vi "Lab Panel V4.89.vi"() -> ()   [LabVIEW 2013] (continued)
                              tunnel: w5371 -> [_ w5375]
                              frame False {
                              }
                              frame True {
                                n2890 = Concatenate Strings("LA02-2 ", w5375) -> (w5378:string)
                                n2891 = One Button Dialog(message=w5378) -> ()  [unwired: 1 in, 1 out]
                              }
                            }
                          }
                          frame #4 {
                            n2892 = Greater?(x=w5380, y=w5383) -> (0:w5382:bool)
                            n2893 = case shown="True" w5382 {
                              tunnel: [w5384 0] -> w5379
                              tunnel: w5380 -> [w5384 _]
                              tunnel: w5381 -> [_ w5385]
                              frame False {
                              }
                              frame True {
                                n2894 = Concatenate Strings("LA03-1 ", w5385) -> (w5388:string)
                                n2895 = One Button Dialog(message=w5388) -> ()  [unwired: 1 in, 1 out]
                              }
                            }
                          }
                          frame #5 {
                            n2896 = Greater?(x=w5389, y=w5393) -> (0:w5392:bool)
                            n2897 = case shown="True" w5392 {
                              tunnel: [w5394 0] -> w5390
                              tunnel: w5389 -> [w5394 _]
                              tunnel: w5391 -> [_ w5395]
                              frame False {
                              }
                              frame True {
                                n2898 = Concatenate Strings("LA03-2 ", w5395) -> (w5398:string)
                                n2899 = One Button Dialog(message=w5398) -> ()  [unwired: 1 in, 1 out]
                              }
                            }
                          }
                          frame #6 {
                            n2900 = Greater?(x=w5400, y=w5403) -> (0:w5402:bool)
                            n2901 = case shown="True" w5402 {
                              tunnel: [w5404 0] -> w5399
                              tunnel: w5400 -> [w5404 _]
                              tunnel: w5401 -> [_ w5405]
                              frame False {
                              }
                              frame True {
                                n2902 = Concatenate Strings("LA04-1 ", w5405) -> (w5408:string)
                                n2903 = One Button Dialog(message=w5408) -> ()  [unwired: 1 in, 1 out]
                              }
                            }
                          }
                          frame #7 {
                            n2904 = Greater?(x=w5410, y=w5413) -> (0:w5412:bool)
                            n2905 = case shown="True" w5412 {
                              tunnel: [w5414 0] -> w5409
                              tunnel: w5410 -> [w5414 _]
                              tunnel: w5411 -> [_ w5415]
                              frame False {
                              }
                              frame True {
                                n2906 = Concatenate Strings("LA04-2 ", w5415) -> (w5418:string)
                                n2907 = One Button Dialog(message=w5418) -> ()  [unwired: 1 in, 1 out]
                              }
                            }
                          }
                          frame #8 {
                            n2908 = Greater?(x=w5420, y=w5423) -> (0:w5422:bool)
                            n2909 = case shown="True" w5422 {
                              tunnel: [w5424 0] -> w5419
                              tunnel: w5420 -> [w5424 _]
                              tunnel: w5421 -> [_ w5425]
                              frame False {
                              }
                              frame True {
                                n2910 = Concatenate Strings("LA05-1 ", w5425) -> (w5428:string)
                                n2911 = One Button Dialog(message=w5428) -> ()  [unwired: 1 in, 1 out]
                              }
                            }
                          }
                          frame #9 {
                            n2912 = Greater?(x=w5430, y=w5433) -> (0:w5432:bool)
                            n2913 = case shown="True" w5432 {
                              tunnel: [w5434 0] -> w5429
                              tunnel: w5430 -> [w5434 _]
                              tunnel: w5431 -> [_ w5435]
                              frame False {
                              }
                              frame True {
                                n2914 = Concatenate Strings("LA05-2 ", w5435) -> (w5438:string)
                                n2915 = One Button Dialog(message=w5438) -> ()  [unwired: 1 in, 1 out]
                              }
                            }
                          }
                        }
                        n2916 = Bundle By Name(cluster=w5337, "LAB01-1"=w5335, "LAB01-2"=w5333, "LAB02-1"=w5330, "LAB02-2"=w5327, "LAB03-1"=w5325, "LAB03-2"=w5324, "LAB04-1"=w5321, "LAB04-2"=w5319, "LAB05-1"=w5317, "LAB05-2"=w5315) -> (w5336:T8)
                        n2917 = local write "JIG RELAY CYCLES"(w5336) -> ()
                      }
                    }
                  }
                }
              }
            }
          }
          frame #19 {
            # "get temperature values"
            n2918 = local read "PANEL #"() -> (w5439:dbl)
            n2919 = local read "simulate"() -> (w5452:bool)
            n2920 = local read "Temp Test Cal"() -> (w5449:dbl)
            n2921 = stacked-sequence {
              seq-local: [w5453 _] -> [_ w5491]
              tunnel: w5452 -> [_ w5505]
              tunnel: T14 {"1  (A) cal"=1.0, "1 (V) cal"=1.0, "1 (PF) cal"=1.0, "1 (TL) cal"=1.0, "1 (TN) cal"=1.0, "2 (A) cal"=1.0, "2 (V) cal"=1.0, "2 (PF) cal"=1.0, "2 (TL) cal"=1.0, "2 (TN) cal"=1.0} ("CAL LAB01") -> [_ w5504]
              tunnel: w5450 -> [_ w5503]
              tunnel: w5449 -> [_ w5502]
              tunnel: w5448 -> [_ w5501]
              tunnel: w5447 -> [_ w5500]
              tunnel: w5446 -> [_ w5499]
              tunnel: w5445 -> [_ w5498]
              tunnel: w5444 -> [_ w5497]
              tunnel: w5443 -> [_ w5496]
              tunnel: w5442 -> [_ w5495]
              tunnel: w5441 -> [_ w5494]
              tunnel: w5440 -> [_ w5493]
              tunnel: w5439 -> [_ w5492]
              frame #0 {
                n2922 = local read "Select COM port"() -> (w5456:refnum<visa-resource-name>)
                "COM port" <- w5456
                n2923 = global write "Global 1.vi" "tmp dly lps"("Temp Delay Lps") -> ()
                n2924 = global write "Global 1.vi" "dly value"("Temp Value") -> ()
                n2925 = global write "Global 1.vi" "COM port"(w5456) -> ()
                n2926 = local read "jig cycle"() -> (w5458:dbl)
                n2927 = local read "on loops"() -> (w5460:dbl)
                n2928 = Add(x=w5460, y=3) -> (x+y=w5461:dbl)
                n2929 = local read "PANEL #"() -> (w5457:dbl)
                n2930 = Equal?(x=w5458, y=w5461) -> (x = y?=w5453:bool)
                n2931 = case shown="True" w5453 {
                  tunnel: w5457 -> [_ w5465]
                  frame False {
                  }
                  frame True {
                    n2932 = local read "simulate"() -> (w5462:bool)
                    n2933 = case shown="1" w5465 {
                      tunnel: 1.0 -> [_ w5470 w5472 w5478 w5482 w5487]
                      tunnel: w5462 -> [_ w5466 w5471 w5476 w5483 w5486]
                      frame 0, Default {
                      }
                      frame 1 {
                        w5468 = FALSE
                        n2934 = call "sub vi - GET ALL TEMP v6.vi"("LA01-EN"=TRUE, "simulate"=w5466, "LA02-EN"=w5468, "LA03-EN"=w5468, "LA04-EN"=w5468, "LA05-EN"=w5468, "Gen Cal Value"=w5470) -> ("LA01 TEMP"=w5467:T24)  [unwired: 3 in, 5 out]
                        n2935 = local write "LAB01 TEMP"(w5467) -> ()
                      }
                      frame 2 {
                        w5473 = FALSE
                        n2936 = call "sub vi - GET ALL TEMP v6.vi"("LA01-EN"=w5473, "simulate"=w5471, "LA02-EN"=TRUE, "LA03-EN"=w5473, "LA04-EN"=w5473, "LA05-EN"=w5473, "Gen Cal Value"=w5472) -> ("LA02 TEMP"=w5475:T24)  [unwired: 3 in, 5 out]
                        n2937 = local write "LAB02 TEMP"(w5475) -> ()
                      }
                      frame 3 {
                        w5479 = FALSE
                        n2938 = call "sub vi - GET ALL TEMP v6.vi"("LA01-EN"=w5479, "simulate"=w5476, "LA02-EN"=w5479, "LA03-EN"=TRUE, "LA04-EN"=w5479, "LA05-EN"=w5479, "Gen Cal Value"=w5478) -> ("LA03 TEMP"=w5477:T24)  [unwired: 3 in, 5 out]
                        n2939 = local write "LAB03 TEMP"(w5477) -> ()
                      }
                      frame 4 {
                        w5484 = FALSE
                        n2940 = call "sub vi - GET ALL TEMP v6.vi"("LA01-EN"=w5484, "simulate"=w5483, "LA02-EN"=w5484, "LA03-EN"=w5484, "LA04-EN"=TRUE, "LA05-EN"=w5484, "Gen Cal Value"=w5482) -> ("LA04 TEMP"=w5481:T24)  [unwired: 3 in, 5 out]
                        n2941 = local write "LAB04 TEMP"(w5481) -> ()
                      }
                      frame 5 {
                        w5489 = FALSE
                        n2942 = call "sub vi - GET ALL TEMP v6.vi"("LA01-EN"=w5489, "simulate"=w5486, "LA02-EN"=w5489, "LA03-EN"=w5489, "LA04-EN"=w5489, "LA05-EN"=TRUE, "Gen Cal Value"=w5487) -> ("LA05 TEMP"=w5488:T24)  [unwired: 3 in, 5 out]
                        n2943 = local write "LAB05 TEMP"(w5488) -> ()
                      }
                    }
                    n2944 = local write "TEMP"(TRUE) -> ()
                  }
                }
              }
              frame #1 {
                n2945 = case shown="True" w5491 {
                  tunnel: w5505 -> [_ w5519]
                  tunnel: w5504 -> [_ w5518]
                  tunnel: w5503 -> [_ w5517]
                  tunnel: w5502 -> [_ w5516]
                  tunnel: w5501 -> [_ w5515]
                  tunnel: w5500 -> [_ w5514]
                  tunnel: w5499 -> [_ w5513]
                  tunnel: w5498 -> [_ w5512]
                  tunnel: w5497 -> [_ w5511]
                  tunnel: w5496 -> [_ w5510]
                  tunnel: w5495 -> [_ w5509]
                  tunnel: w5494 -> [_ w5508]
                  tunnel: w5493 -> [_ w5507]
                  tunnel: w5492 -> [_ w5506]
                  frame False {
                  }
                  frame True {
                    n2946 = case shown="1" w5506 {
                      tunnel: w5519 -> [_ w5532 w5577 w5622 w5667 w5712]
                      tunnel: w5518 -> [_ w5531 w5576 w5621 w5666 w5711]
                      tunnel: w5517 -> [_ w5529 _ _ _ _]
                      tunnel: w5516 -> [_ w5525 w5575 w5620 w5665 w5710]
                      tunnel: w5515 -> [_ w5520 _ _ _ _]
                      tunnel: w5514 -> [_ _ w5566 _ _ _]
                      tunnel: w5513 -> [_ _ w5565 _ _ _]
                      tunnel: w5512 -> [_ _ _ w5611 _ _]
                      tunnel: w5511 -> [_ _ _ w5610 _ _]
                      tunnel: w5510 -> [_ _ _ _ w5656 _]
                      tunnel: w5509 -> [_ _ _ _ w5655 _]
                      tunnel: w5508 -> [_ _ _ _ _ w5701]
                      tunnel: w5507 -> [_ _ _ _ _ w5700]
                      frame ..0 {
                      }
                      frame 1 {
                        n2947 = case shown="False" w5532 {
                          tunnel: [w5563 w5564] -> w5548
                          tunnel: w5531 -> [_ w5564]
                          frame False {
                            n2948 = local read "CAL LAB01"() -> (w5563:T14)
                          }
                          frame True {
                          }
                        }
                        n2949 = local read "LAB01 TEMP"() -> (w5538:T12)
                        n2950 = local read "TEMP LA01"() -> (w5539:T9)
                        n2951 = call "sub vi - temperature delay v2.vi"("temp values IN"=w5539, "temp signals"=w5538) -> ("T2-N"=w5534:dbl, "T2-L"=w5535:dbl, "T1-N"=w5536:dbl, "T1-L"=w5537:dbl, "temp values OUT"=w5533:T43)  [unwired: 5 in]
                        n2952 = Unbundle By Name(w5548) -> ("1 (TL) cal"=w5543:dbl, "1 (TN) cal"=w5542:dbl, "2 (TL) cal"=w5541:dbl, "2 (TN) cal"=w5540:dbl)  [unwired: 6 out]
                        n2953 = local write "TEMP LA01"(w5533) -> ()
                        n2954 = Multiply(x=w5537, y=w5543) -> (x*y=w5530:dbl)
                        n2955 = Multiply(x=w5536, y=w5542) -> (x*y=w5527:dbl)
                        n2956 = Multiply(x=w5535, y=w5541) -> (x*y=w5524:dbl)
                        n2957 = Multiply(x=w5534, y=w5540) -> (x*y=w5523:dbl)
                        n2958 = case shown="True" w5529 {
                          tunnel: w5530 -> [w5557 w5562]
                          tunnel: w5525 -> [_ w5560]
                          tunnel: [w5557 w5561] -> w5528
                          tunnel: w5527 -> [w5556 w5559]
                          tunnel: [w5556 w5558] -> w5526
                          frame False {
                          }
                          frame True {
                            n2959 = Multiply(x=w5560, y=w5559) -> (x*y=w5558:dbl)
                            n2960 = Multiply(x=w5560, y=w5562) -> (x*y=w5561:dbl)
                          }
                        }
                        n2961 = case shown="True" w5520 {
                          tunnel: w5524 -> [w5550 w5555]
                          tunnel: w5525 -> [_ w5553]
                          tunnel: [w5550 w5554] -> w5522
                          tunnel: w5523 -> [w5549 w5552]
                          tunnel: [w5549 w5551] -> w5521
                          frame False {
                          }
                          frame True {
                            n2962 = Multiply(x=w5553, y=w5552) -> (x*y=w5551:dbl)
                            n2963 = Multiply(x=w5553, y=w5555) -> (x*y=w5554:dbl)
                          }
                        }
                        n2964 = local read "SIG LAB01-2"() -> (w5545:T2)
                        n2965 = local read "SIG LAB01-1"() -> (w5547:T2)
                        n2966 = Bundle By Name(cluster=w5547, "Tmp Live"=w5528, "Tmp Neut"=w5526) -> (w5546:T2)
                        n2967 = Bundle By Name(cluster=w5545, "Tmp Live"=w5522, "Tmp Neut"=w5521) -> (w5544:T2)
                        n2968 = local write "SIG LAB01-1"(w5546) -> ()
                        n2969 = local write "SIG LAB01-2"(w5544) -> ()
                      }
                      frame 2 {
                        n2970 = case shown="True" w5577 {
                          tunnel: [w5608 w5609] -> w5593
                          tunnel: w5576 -> [_ w5609]
                          frame False {
                            n2971 = local read "CAL LAB02"() -> (w5608:T15)
                          }
                          frame True {
                          }
                        }
                        n2972 = local read "LAB02 TEMP"() -> (w5584:T12)
                        n2973 = local read "TEMP LA02"() -> (w5583:T9)
                        n2974 = call "sub vi - temperature delay v2.vi"("temp values IN"=w5583, "temp signals"=w5584) -> ("T2-N"=w5578:dbl, "T2-L"=w5579:dbl, "T1-N"=w5580:dbl, "T1-L"=w5581:dbl, "temp values OUT"=w5582:T43)  [unwired: 5 in]
                        n2975 = Unbundle By Name(w5593) -> ("1 (TL) cal"=w5588:dbl, "1 (TN) cal"=w5587:dbl, "2 (TL) cal"=w5586:dbl, "2 (TN) cal"=w5585:dbl)  [unwired: 6 out]
                        n2976 = local write "TEMP LA02"(w5582) -> ()
                        n2977 = Multiply(x=w5581, y=w5588) -> (x*y=w5574:dbl)
                        n2978 = Multiply(x=w5580, y=w5587) -> (x*y=w5573:dbl)
                        n2979 = Multiply(x=w5579, y=w5586) -> (x*y=w5570:dbl)
                        n2980 = Multiply(x=w5578, y=w5585) -> (x*y=w5569:dbl)
                        n2981 = case shown="True" w5566 {
                          tunnel: w5574 -> [w5602 w5607]
                          tunnel: w5575 -> [_ w5605]
                          tunnel: [w5602 w5606] -> w5572
                          tunnel: w5573 -> [w5601 w5604]
                          tunnel: [w5601 w5603] -> w5571
                          frame False {
                          }
                          frame True {
                            n2982 = Multiply(x=w5605, y=w5604) -> (x*y=w5603:dbl)
                            n2983 = Multiply(x=w5605, y=w5607) -> (x*y=w5606:dbl)
                          }
                        }
                        n2984 = case shown="True" w5565 {
                          tunnel: w5570 -> [w5595 w5600]
                          tunnel: w5575 -> [_ w5598]
                          tunnel: [w5595 w5599] -> w5568
                          tunnel: w5569 -> [w5594 w5597]
                          tunnel: [w5594 w5596] -> w5567
                          frame False {
                          }
                          frame True {
                            n2985 = Multiply(x=w5598, y=w5597) -> (x*y=w5596:dbl)
                            n2986 = Multiply(x=w5598, y=w5600) -> (x*y=w5599:dbl)
                          }
                        }
                        n2987 = local read "SIG LAB02-2"() -> (w5590:T2)
                        n2988 = local read "SIG LAB02-1"() -> (w5592:T2)
                        n2989 = Bundle By Name(cluster=w5592, "Tmp Live"=w5572, "Tmp Neut"=w5571) -> (w5591:T2)
                        n2990 = Bundle By Name(cluster=w5590, "Tmp Live"=w5568, "Tmp Neut"=w5567) -> (w5589:T2)
                        n2991 = local write "SIG LAB02-1"(w5591) -> ()
                        n2992 = local write "SIG LAB02-2"(w5589) -> ()
                      }
                      frame 3 {
                        n2993 = case shown="False" w5622 {
                          tunnel: [w5653 w5654] -> w5638
                          tunnel: w5621 -> [_ w5654]
                          frame False {
                            n2994 = local read "CAL LAB03"() -> (w5653:T14)
                          }
                          frame True {
                          }
                        }
                        n2995 = local read "TEMP LA03"() -> (w5628:T9)
                        n2996 = local read "LAB03 TEMP"() -> (w5629:T12)
                        n2997 = call "sub vi - temperature delay v2.vi"("temp values IN"=w5628, "temp signals"=w5629) -> ("T2-N"=w5623:dbl, "T2-L"=w5624:dbl, "T1-N"=w5625:dbl, "T1-L"=w5626:dbl, "temp values OUT"=w5627:T43)  [unwired: 5 in]
                        n2998 = Unbundle By Name(w5638) -> ("1 (TL) cal"=w5633:dbl, "1 (TN) cal"=w5632:dbl, "2 (TL) cal"=w5631:dbl, "2 (TN) cal"=w5630:dbl)  [unwired: 6 out]
                        n2999 = local write "TEMP LA03"(w5627) -> ()
                        n3000 = Multiply(x=w5626, y=w5633) -> (x*y=w5619:dbl)
                        n3001 = Multiply(x=w5625, y=w5632) -> (x*y=w5618:dbl)
                        n3002 = Multiply(x=w5624, y=w5631) -> (x*y=w5615:dbl)
                        n3003 = Multiply(x=w5623, y=w5630) -> (x*y=w5614:dbl)
                        n3004 = case shown="True" w5610 {
                          tunnel: w5615 -> [w5640 w5645]
                          tunnel: w5620 -> [_ w5643]
                          tunnel: [w5640 w5644] -> w5613
                          tunnel: w5614 -> [w5639 w5642]
                          tunnel: [w5639 w5641] -> w5612
                          frame False {
                          }
                          frame True {
                            n3005 = Multiply(x=w5643, y=w5642) -> (x*y=w5641:dbl)
                            n3006 = Multiply(x=w5643, y=w5645) -> (x*y=w5644:dbl)
                          }
                        }
                        n3007 = case shown="True" w5611 {
                          tunnel: w5619 -> [w5647 w5652]
                          tunnel: w5620 -> [_ w5650]
                          tunnel: [w5647 w5651] -> w5617
                          tunnel: w5618 -> [w5646 w5649]
                          tunnel: [w5646 w5648] -> w5616
                          frame False {
                          }
                          frame True {
                            n3008 = Multiply(x=w5650, y=w5649) -> (x*y=w5648:dbl)
                            n3009 = Multiply(x=w5650, y=w5652) -> (x*y=w5651:dbl)
                          }
                        }
                        n3010 = local read "SIG LAB03-2"() -> (w5635:T2)
                        n3011 = local read "SIG LAB03-1"() -> (w5637:T2)
                        n3012 = Bundle By Name(cluster=w5637, "Tmp Live"=w5617, "Tmp Neut"=w5616) -> (w5636:T2)
                        n3013 = Bundle By Name(cluster=w5635, "Tmp Live"=w5613, "Tmp Neut"=w5612) -> (w5634:T2)
                        n3014 = local write "SIG LAB03-1"(w5636) -> ()
                        n3015 = local write "SIG LAB03-2"(w5634) -> ()
                      }
                      frame 4 {
                        n3016 = case shown="False" w5667 {
                          tunnel: [w5698 w5699] -> w5683
                          tunnel: w5666 -> [_ w5699]
                          frame False {
                            n3017 = local read "CAL LAB04"() -> (w5698:T14)
                          }
                          frame True {
                          }
                        }
                        n3018 = local read "LAB04 TEMP"() -> (w5673:T12)
                        n3019 = local read "TEMP LA04"() -> (w5674:T9)
                        n3020 = call "sub vi - temperature delay v2.vi"("temp values IN"=w5674, "temp signals"=w5673) -> ("T2-N"=w5668:dbl, "T2-L"=w5669:dbl, "T1-N"=w5670:dbl, "T1-L"=w5671:dbl, "temp values OUT"=w5672:T43)  [unwired: 5 in]
                        n3021 = Unbundle By Name(w5683) -> ("1 (TL) cal"=w5678:dbl, "1 (TN) cal"=w5677:dbl, "2 (TL) cal"=w5676:dbl, "2 (TN) cal"=w5675:dbl)  [unwired: 6 out]
                        n3022 = local write "TEMP LA04"(w5672) -> ()
                        n3023 = Multiply(x=w5671, y=w5678) -> (x*y=w5664:dbl)
                        n3024 = Multiply(x=w5670, y=w5677) -> (x*y=w5663:dbl)
                        n3025 = Multiply(x=w5669, y=w5676) -> (x*y=w5660:dbl)
                        n3026 = Multiply(x=w5668, y=w5675) -> (x*y=w5659:dbl)
                        n3027 = case shown="True" w5655 {
                          tunnel: w5660 -> [w5685 w5690]
                          tunnel: w5665 -> [_ w5688]
                          tunnel: [w5685 w5689] -> w5658
                          tunnel: w5659 -> [w5684 w5687]
                          tunnel: [w5684 w5686] -> w5657
                          frame False {
                          }
                          frame True {
                            n3028 = Multiply(x=w5688, y=w5687) -> (x*y=w5686:dbl)
                            n3029 = Multiply(x=w5688, y=w5690) -> (x*y=w5689:dbl)
                          }
                        }
                        n3030 = case shown="True" w5656 {
                          tunnel: w5664 -> [w5692 w5697]
                          tunnel: w5665 -> [_ w5695]
                          tunnel: [w5692 w5696] -> w5662
                          tunnel: w5663 -> [w5691 w5694]
                          tunnel: [w5691 w5693] -> w5661
                          frame False {
                          }
                          frame True {
                            n3031 = Multiply(x=w5695, y=w5694) -> (x*y=w5693:dbl)
                            n3032 = Multiply(x=w5695, y=w5697) -> (x*y=w5696:dbl)
                          }
                        }
                        n3033 = local read "SIG LAB04-2"() -> (w5680:T2)
                        n3034 = local read "SIG LAB04-1"() -> (w5682:T2)
                        n3035 = Bundle By Name(cluster=w5682, "Tmp Live"=w5662, "Tmp Neut"=w5661) -> (w5681:T2)
                        n3036 = Bundle By Name(cluster=w5680, "Tmp Live"=w5658, "Tmp Neut"=w5657) -> (w5679:T2)
                        n3037 = local write "SIG LAB04-1"(w5681) -> ()
                        n3038 = local write "SIG LAB04-2"(w5679) -> ()
                      }
                      frame 5.. {
                        n3039 = case shown="False" w5712 {
                          tunnel: [w5743 w5744] -> w5728
                          tunnel: w5711 -> [_ w5744]
                          frame False {
                            n3040 = local read "CAL LAB05"() -> (w5743:T14)
                          }
                          frame True {
                          }
                        }
                        n3041 = local read "LAB05 TEMP"() -> (w5718:T12)
                        n3042 = local read "TEMP LA05"() -> (w5719:T9)
                        n3043 = call "sub vi - temperature delay v2.vi"("temp values IN"=w5719, "temp signals"=w5718) -> ("T2-N"=w5714:dbl, "T2-L"=w5715:dbl, "T1-N"=w5716:dbl, "T1-L"=w5717:dbl, "temp values OUT"=w5713:T43)  [unwired: 5 in]
                        n3044 = local write "TEMP LA05"(w5713) -> ()
                        n3045 = Unbundle By Name(w5728) -> ("1 (TL) cal"=w5720:dbl, "1 (TN) cal"=w5723:dbl, "2 (TL) cal"=w5722:dbl, "2 (TN) cal"=w5721:dbl)  [unwired: 6 out]
                        n3046 = Multiply(x=w5717, y=w5720) -> (x*y=w5709:dbl)
                        n3047 = Multiply(x=w5716, y=w5723) -> (x*y=w5708:dbl)
                        n3048 = Multiply(x=w5715, y=w5722) -> (x*y=w5705:dbl)
                        n3049 = Multiply(x=w5714, y=w5721) -> (x*y=w5704:dbl)
                        n3050 = case shown="True" w5700 {
                          tunnel: w5705 -> [w5730 w5735]
                          tunnel: w5710 -> [_ w5733]
                          tunnel: [w5730 w5734] -> w5703
                          tunnel: w5704 -> [w5729 w5732]
                          tunnel: [w5729 w5731] -> w5702
                          frame False {
                          }
                          frame True {
                            n3051 = Multiply(x=w5733, y=w5732) -> (x*y=w5731:dbl)
                            n3052 = Multiply(x=w5733, y=w5735) -> (x*y=w5734:dbl)
                          }
                        }
                        n3053 = case shown="True" w5701 {
                          tunnel: w5709 -> [w5737 w5742]
                          tunnel: w5710 -> [_ w5740]
                          tunnel: [w5737 w5741] -> w5707
                          tunnel: w5708 -> [w5736 w5739]
                          tunnel: [w5736 w5738] -> w5706
                          frame False {
                          }
                          frame True {
                            n3054 = Multiply(x=w5740, y=w5739) -> (x*y=w5738:dbl)
                            n3055 = Multiply(x=w5740, y=w5742) -> (x*y=w5741:dbl)
                          }
                        }
                        n3056 = local read "SIG LAB05-1"() -> (w5727:T2)
                        n3057 = Bundle By Name(cluster=w5727, "Tmp Live"=w5707, "Tmp Neut"=w5706) -> (w5726:T2)
                        n3058 = local read "SIG LAB05-2"() -> (w5725:T2)
                        n3059 = Bundle By Name(cluster=w5725, "Tmp Live"=w5703, "Tmp Neut"=w5702) -> (w5724:T2)
                        n3060 = local write "SIG LAB05-1"(w5726) -> ()
                        n3061 = local write "SIG LAB05-2"(w5724) -> ()
                      }
                    }
                  }
                }
              }
            }
          }
          frame #20 {
            # "write data to display panel"
            n3062 = global write "Global display 1.vi" "TEST 5-2"(w5779) -> ()
            n3063 = global write "Global display 1.vi" "TEST 4-2"(w5781) -> ()
            n3064 = global write "Global display 1.vi" "TEST 1-2"(w5787) -> ()
            n3065 = global write "Global display 1.vi" "TEST 3-1"(w5784) -> ()
            n3066 = global write "Global display 1.vi" "TEST 5-1"(w5780) -> ()
            n3067 = global write "Global display 1.vi" "TEST 1-1"(w5788) -> ()
            n3068 = global write "Global display 1.vi" "TEST 3-2"(w5783) -> ()
            n3069 = global write "Global display 1.vi" "TEST 4-1"(w5782) -> ()
            n3070 = global write "Global display 1.vi" "TEST 2-2"(w5785) -> ()
            n3071 = global write "Global display 1.vi" "TEST 2-1"(w5786) -> ()
            n3072 = global read "Global display 3.vi" "log 1-1"() -> (→"LOG LAB01-1":string)
            n3073 = global read "Global display 3.vi" "log 3-1"() -> (→"LOG LAB03-1":string)
            n3074 = global read "Global display 3.vi" "log 1-2"() -> (→"LOG LAB01-2":string)
            n3075 = property on="Tab Control 2" class="TabCtl (strict)"() -> ("Pages"=w5778:refnum<vi>[])  [unwired: 2 in, 2 out]
            n3076 = global read "Global display 3.vi" "log 2-1"() -> (→"LOG LAB02-1":string)
            n3077 = global read "Global display 3.vi" "log 2-2"() -> (→"LOG LAB02-2":string)
            n3078 = global read "Global display 3.vi" "log 4-2"() -> (→"LOG LAB04-2":string)
            n3079 = global read "Global display 3.vi" "log 5-2"() -> (→"LOG LAB05-2":string)
            n3080 = global read "Global display 3.vi" "log 5-1"() -> (→"LOG LAB05-1":string)
            n3081 = global read "Global display 3.vi" "log 4-1"() -> (→"LOG LAB04-1":string)
            n3082 = global read "Global display 3.vi" "log 3-2"() -> (→"LOG LAB03-2":string)
            n3083 = Index Array(array=w5778, index=8) -> (element=w5776:refnum<vi>)
            n3084 = property class="Page"(reference=w5776) -> ("PageVis"=w5775:bool)  [unwired: 1 in, 2 out]
            n3085 = global write "Global display 3.vi" "admin"(w5775) -> ()
            n3086 = local read "O/I  LAB05-2"() -> (w5829:bool)
            n3087 = local read "O/I  LAB05-1"() -> (w5830:bool)
            n3088 = local read "O/I  LAB03-2"() -> (w5833:bool)
            n3089 = local read "O/I  LAB04-2"() -> (w5831:bool)
            n3090 = local read "O/I  LAB04-1"() -> (w5832:bool)
            n3091 = local read "O/I  LAB03-1"() -> (w5834:bool)
            n3092 = local read "O/I  LAB01-2"() -> (w5837:bool)
            n3093 = local read "O/I  LAB01-1"() -> (w5838:bool)
            n3094 = local read "O/I  LAB02-1"() -> (w5836:bool)
            n3095 = local read "O/I  LAB02-2"() -> (w5835:bool)
            n3096 = global write "Global display 1.vi" "5-2 O/F"(w5829) -> ()
            n3097 = global write "Global display 1.vi" "5-1 O/F"(w5830) -> ()
            n3098 = global write "Global display 1.vi" "4-1 O/F"(w5832) -> ()
            n3099 = global write "Global display 1.vi" "4-2 O/F"(w5831) -> ()
            n3100 = global write "Global display 1.vi" "3-2 O/F"(w5833) -> ()
            n3101 = global write "Global display 1.vi" "3-1 O/F"(w5834) -> ()
            n3102 = global write "Global display 1.vi" "2-2 O/F"(w5835) -> ()
            n3103 = global write "Global display 1.vi" "2-1 O/F"(w5836) -> ()
            n3104 = global write "Global display 1.vi" "1-2 O/F"(w5837) -> ()
            n3105 = global write "Global display 1.vi" "1-1 O/F"(w5838) -> ()
            n3106 = local read "TEMP START LAB02-2"() -> (w5761:cluster{"TL":dbl, "TN":dbl})
            n3107 = local read "run lab05-2"() -> (w5819:bool)
            n3108 = local read "TEMP START LAB01-2"() -> (w5763:cluster{"TL":dbl, "TN":dbl})
            n3109 = local read "TEMP START LAB02-1"() -> (w5762:cluster{"TL":dbl, "TN":dbl})
            n3110 = local read "TEMP START LAB04-1"() -> (w5758:cluster{"TL":dbl, "TN":dbl})
            n3111 = local read "TEMP START LAB04-2"() -> (w5757:cluster{"TL":dbl, "TN":dbl})
            n3112 = local read "run lab04-1"() -> (w5822:bool)
            n3113 = local read "run lab04-2"() -> (w5821:bool)
            n3114 = local read "run lab05-1"() -> (w5820:bool)
            n3115 = local read "TEMP START LAB01-1"() -> (w5764:cluster{"TL":dbl, "TN":dbl})
            n3116 = local read "TEMP START LAB05-2"() -> (w5755:cluster{"TL":dbl, "TN":dbl})
            n3117 = local read "TEMP START LAB05-1"() -> (w5756:cluster{"TL":dbl, "TN":dbl})
            n3118 = local read "run lab03-2"() -> (w5823:bool)
            n3119 = local read "TEMP START LAB03-2"() -> (w5759:cluster{"TL":dbl, "TN":dbl})
            n3120 = local read "TEMP START LAB03-1"() -> (w5760:cluster{"TL":dbl, "TN":dbl})
            n3121 = local read "run lab02-1"() -> (w5826:bool)
            n3122 = local read "run lab03-1"() -> (w5824:bool)
            n3123 = local read "run lab01-2"() -> (w5827:bool)
            n3124 = local read "run lab02-2"() -> (w5825:bool)
            n3125 = local read "run lab01-1"() -> (w5828:bool)
            n3126 = global write "Global display 1.vi" "5-2 R/S"(w5819) -> ()
            n3127 = global write "Global display 1.vi" "5-1 R/S"(w5820) -> ()
            n3128 = global write "Global display 1.vi" "4-2 R/S"(w5821) -> ()
            n3129 = global write "Global display 1.vi" "4-1 R/S"(w5822) -> ()
            n3130 = global write "Global display 1.vi" "3-2 R/S"(w5823) -> ()
            n3131 = global write "Global display 1.vi" "1-2 R/S"(w5827) -> ()
            n3132 = global write "Global display 1.vi" "2-1 R/S"(w5826) -> ()
            n3133 = global write "Global display 1.vi" "3-1 R/S"(w5824) -> ()
            n3134 = global write "Global display 1.vi" "2-2 R/S"(w5825) -> ()
            n3135 = global write "Global display 1.vi" "1-1 R/S"(w5828) -> ()
            n3136 = global write "Global display 3.vi" "TEMP ST 05-2"(w5755) -> ()
            n3137 = global write "Global display 3.vi" "TEMP ST 05-1"(w5756) -> ()
            n3138 = global write "Global display 3.vi" "TEMP ST 03-2"(w5759) -> ()
            n3139 = global write "Global display 3.vi" "TEMP ST 04-2"(w5757) -> ()
            n3140 = global write "Global display 3.vi" "TEMP ST 01-1"(w5764) -> ()
            n3141 = global write "Global display 3.vi" "TEMP ST 01-2"(w5763) -> ()
            n3142 = global write "Global display 3.vi" "TEMP ST 04-1"(w5758) -> ()
            n3143 = global write "Global display 3.vi" "TEMP ST 02-1"(w5762) -> ()
            n3144 = global write "Global display 3.vi" "TEMP ST 02-2"(w5761) -> ()
            n3145 = global write "Global display 3.vi" "TEMP ST 03-1"(w5760) -> ()
            n3146 = local read "DISP LAB04-2"() -> (w5811:T4)
            n3147 = local read "DISP LAB05-1"() -> (w5810:T4)
            n3148 = local read "DISP LAB04-1"() -> (w5812:T4)
            n3149 = local read "DISP LAB05-2"() -> (w5809:T4)
            n3150 = local read "DISP LAB03-1"() -> (w5814:T4)
            n3151 = local read "DISP LAB03-2"() -> (w5813:T4)
            n3152 = local read "DISP LAB01-2"() -> (w5817:T4)
            n3153 = local read "DISP LAB02-1"() -> (w5816:T4)
            n3154 = local read "DISP LAB02-2"() -> (w5815:T4)
            n3155 = local read "DISP LAB01-1"() -> (w5818:T4)
            n3156 = local read "TEMP RISE LAB05-1"() -> (w5746:cluster{"TL":dbl, "TN":dbl})
            n3157 = local read "TEMP RISE LAB05-2"() -> (w5745:cluster{"TL":dbl, "TN":dbl})
            n3158 = local read "TEMP RISE LAB04-2"() -> (w5747:cluster{"TL":dbl, "TN":dbl})
            n3159 = local read "TEMP RISE LAB04-1"() -> (w5748:cluster{"TL":dbl, "TN":dbl})
            n3160 = local read "TEMP RISE LAB03-2"() -> (w5749:cluster{"TL":dbl, "TN":dbl})
            n3161 = local read "TEMP RISE LAB03-1"() -> (w5750:cluster{"TL":dbl, "TN":dbl})
            n3162 = local read "TEMP RISE LAB01-2"() -> (w5753:cluster{"TL":dbl, "TN":dbl})
            n3163 = local read "TEMP RISE LAB02-2"() -> (w5751:cluster{"TL":dbl, "TN":dbl})
            n3164 = local read "TEMP RISE LAB01-1"() -> (w5754:cluster{"TL":dbl, "TN":dbl})
            n3165 = local read "TEMP RISE LAB02-1"() -> (w5752:cluster{"TL":dbl, "TN":dbl})
            n3166 = global write "Global display 2.vi" "DISP LAB05-1"(w5810) -> ()
            n3167 = global write "Global display 2.vi" "DISP LAB05-2"(w5809) -> ()
            n3168 = global write "Global display 2.vi" "DISP LAB04-2"(w5811) -> ()
            n3169 = global write "Global display 2.vi" "DISP LAB02-1"(w5816) -> ()
            n3170 = global write "Global display 2.vi" "DISP LAB02-2"(w5815) -> ()
            n3171 = global write "Global display 2.vi" "DISP LAB04-1"(w5812) -> ()
            n3172 = global write "Global display 2.vi" "DISP LAB01-2"(w5817) -> ()
            n3173 = global write "Global display 2.vi" "DISP LAB01-1"(w5818) -> ()
            n3174 = global write "Global display 2.vi" "DISP LAB03-1"(w5814) -> ()
            n3175 = global write "Global display 2.vi" "DISP LAB03-2"(w5813) -> ()
            n3176 = global write "Global display 3.vi" "TEMP RS 05-2"(w5745) -> ()
            n3177 = global write "Global display 3.vi" "TEMP RS 05-1"(w5746) -> ()
            n3178 = global write "Global display 3.vi" "TEMP RS 03-2"(w5749) -> ()
            n3179 = global write "Global display 3.vi" "TEMP RS 02-1"(w5752) -> ()
            n3180 = global write "Global display 3.vi" "TEMP RS 02-2"(w5751) -> ()
            n3181 = global write "Global display 3.vi" "TEMP RS 04-2"(w5747) -> ()
            n3182 = global write "Global display 3.vi" "TEMP RS 01-2"(w5753) -> ()
            n3183 = global write "Global display 3.vi" "TEMP RS 03-1"(w5750) -> ()
            n3184 = global write "Global display 3.vi" "TEMP RS 04-1"(w5748) -> ()
            n3185 = global write "Global display 3.vi" "TEMP RS 01-1"(w5754) -> ()
            n3186 = local read "SET LAB05-2"() -> (w5799:T5)
            n3187 = local read "SET LAB05-1"() -> (w5800:T5)
            n3188 = local read "SET LAB04-1"() -> (w5802:T5)
            n3189 = local read "SET LAB04-2"() -> (w5801:T5)
            n3190 = local read "SET LAB03-1"() -> (w5804:T5)
            n3191 = local read "SET LAB03-2"() -> (w5803:T5)
            n3192 = local read "SET LAB02-2"() -> (w5805:T5)
            n3193 = local read "SET LAB01-2"() -> (w5807:T5)
            n3194 = local read "SET LAB02-1"() -> (w5806:T5)
            n3195 = local read "SET LAB01-1"() -> (w5808:T5)
            n3196 = global write "Global display 2.vi" "SET LAB05-2"(w5799) -> ()
            n3197 = global write "Global display 2.vi" "SET LAB05-1"(w5800) -> ()
            n3198 = global write "Global display 2.vi" "SET LAB04-1"(w5802) -> ()
            n3199 = global write "Global display 2.vi" "SET LAB04-2"(w5801) -> ()
            n3200 = global write "Global display 2.vi" "SET LAB03-2"(w5803) -> ()
            n3201 = global write "Global display 2.vi" "SET LAB02-2"(w5805) -> ()
            n3202 = global write "Global display 2.vi" "SET LAB03-1"(w5804) -> ()
            n3203 = global write "Global display 2.vi" "SET LAB01-2"(w5807) -> ()
            n3204 = global write "Global display 2.vi" "SET LAB01-1"(w5808) -> ()
            n3205 = global write "Global display 2.vi" "SET LAB02-1"(w5806) -> ()
            n3206 = local read "RESULT LAB01-1"() -> (w5798:bool)
            n3207 = local read "RESULT LAB03-2"() -> (w5793:bool)
            n3208 = local read "RESULT LAB04-1"() -> (w5792:bool)
            n3209 = local read "RESULT LAB04-2"() -> (w5791:bool)
            n3210 = local read "RESULT LAB02-2"() -> (w5795:bool)
            n3211 = local read "RESULT LAB01-2"() -> (w5797:bool)
            n3212 = local read "RESULT LAB02-1"() -> (w5796:bool)
            n3213 = local read "RESULT LAB03-1"() -> (w5794:bool)
            n3214 = local read "RESULT LAB05-1"() -> (w5790:bool)
            n3215 = local read "RESULT LAB05-2"() -> (w5789:bool)
            n3216 = global write "Global display 2.vi" "RESULT LAB05-1"(w5790) -> ()
            n3217 = global write "Global display 2.vi" "RESULT LAB01-2"(w5797) -> ()
            n3218 = global write "Global display 2.vi" "RESULT LAB03-2"(w5793) -> ()
            n3219 = global write "Global display 2.vi" "RESULT LAB04-1"(w5792) -> ()
            n3220 = global write "Global display 2.vi" "RESULT LAB04-2"(w5791) -> ()
            n3221 = global write "Global display 2.vi" "RESULT LAB05-2"(w5789) -> ()
            n3222 = global write "Global display 2.vi" "RESULT LAB03-1"(w5794) -> ()
            n3223 = global write "Global display 2.vi" "RESULT LAB02-1"(w5796) -> ()
            n3224 = global write "Global display 2.vi" "RESULT LAB02-2"(w5795) -> ()
            n3225 = global write "Global display 2.vi" "RESULT LAB01-1"(w5798) -> ()
          }
          frame #21 {
            # "simulate values"
            n3226 = global write "Global display 4.vi" "LAB deg C"("LAB deg C") -> ()
          }
          frame #22 {
            # "end main and display program"
            n3227 = Quit LabVIEW(quit? (T)="stop all") -> ()
            n3228 = global write "Global display 1.vi" "stop disp"("stop all") -> ()
          }
        }
        n3229 = node-c288() -> ()  [unwired: 1 in, 1 out]
        "loops" <- w309
      }
      n3230 = node-c288(w286) -> ()  [unwired: 1 out]
    }
  }
